vi "DAQmx 9481 Relay (SubVI).vi"(0 "9481 Name":tag="Relay-I", 7 "Relay Control":bool[](array[boolean])=[FALSE, FALSE, FALSE, FALSE], 11 "Error Input":errorcluster, 14 "Stop Program":bool) -> (15 "Relay Error":errorcluster)   [LabVIEW 2011]
uses:
  <vilib>/DAQmx/write.llb/DAQmx Write (Digital 1D Bool NChan 1Samp 1Line).vi
  <vilib>/DAQmx/create/channels.llb/DAQmx Create Channel (DO-Digital Output).vi
  <vilib>/DAQmx/miscellaneous.llb/DAQmx Fill In Error Info.vi
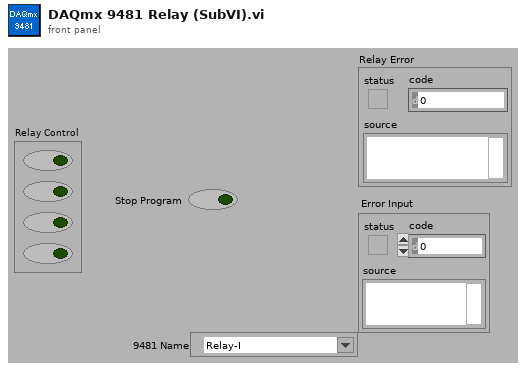
[diagram p1: front panel]
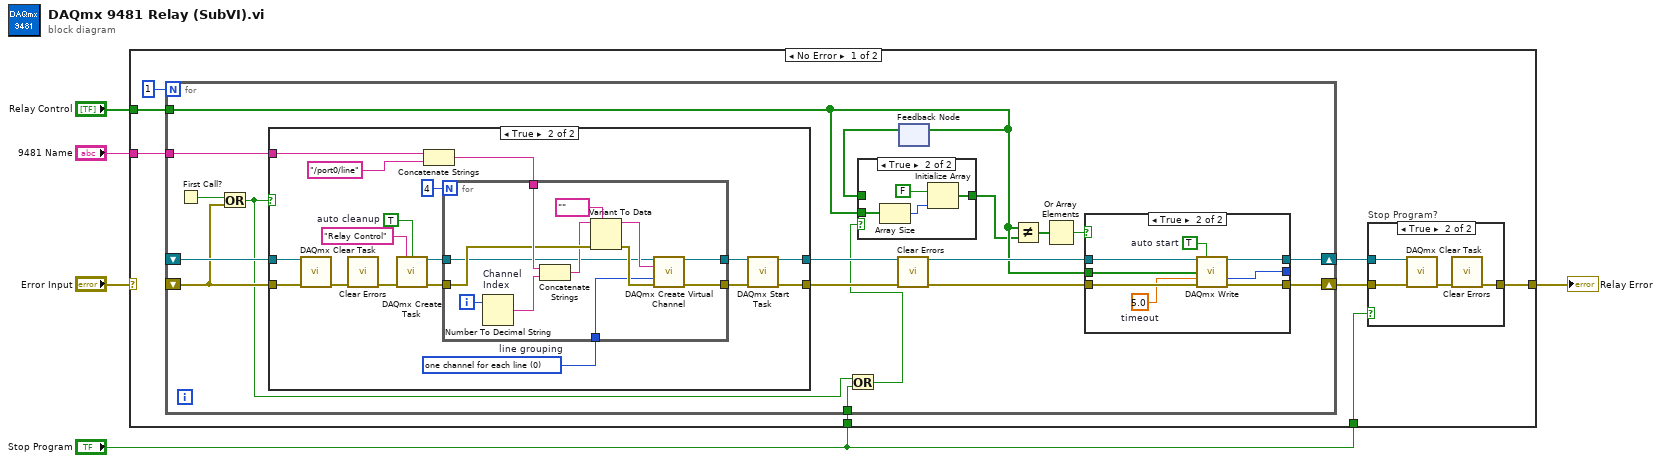
[diagram p0: block diagram]
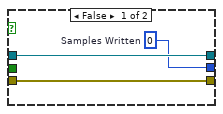
[diagram p3: hidden frame]
diagram:
  n1 = case shown="No Error" "Error Input" {
    selector: "Error Input" -> [_ w83]
    tunnel: "Relay Control" -> [w13 _]
    tunnel: [w12 w83] -> w4
    tunnel: "Stop Program" -> [w9 _]
    tunnel: "9481 Name" -> [w7 _]
    tunnel: "Stop Program" -> [w6 _]
    frame No Error {
      n2 = for {
        N: 1 -> [_]
        tunnel: w13 -> [w29]
        shift-right: [w27] -> w10
        shift-left: _ -> [w26]
        shift-right: [w28] -> w11
        shift-left: _ -> [w17]
        tunnel: w7 -> [w24]
        tunnel: w6 -> [w14]
        n3 = First Call?() -> (First Call?: T/F=w25:bool)
        n4 = Or(x=w25, y=w17) -> (x .or. y?=w16:bool)
        n5 = case shown="True" w16 {
          tunnel: [w48 w54] -> w30
          tunnel: [w47 w53] -> w19
          tunnel: w17 -> [w47 w58]
          tunnel: w26 -> [w48 w59]
          tunnel: w24 -> [_ w52]
          frame False {
          }
          frame True {
            w63 = 0 items=["one channel for each line", "one channel for all lines"]  # line grouping
            w65 = TRUE  # auto cleanup
            n6 = call <vilib>:"DAQmx Clear Task.vi"("task in"=w59, "error in"=w58) -> ("error out"=w57:errorcluster)  [unwired: 13 in]
            n7 = call <vilib>:"Clear Errors.vi"("error in (no error)"=w57) -> ("error out"=w56:errorcluster)  [unwired: 6 in]
            n8 = call <vilib>:"DAQmx Create Task.vi"("new task name"="Relay Control", "auto cleanup"=w65, "error in"=w56) -> ("task out"=w61:refnum<k21>, "error out"=w62:errorcluster)  [unwired: 11 in]
            n9 = Concatenate Strings(w52, "/port0/line" ("string")) -> (w51:string)
            n10 = for {
              N: 4 -> [_]
              tunnel: w51 -> [w75]
              tunnel: w62 -> [w73]
              tunnel: [w67] -> w49
              tunnel: w61 -> [w69]
              tunnel: [w68] -> w50
              tunnel: w63 -> [w66]
              i -> [w76]
              n11 = Number To Decimal String "Channel\nIndex"(number=w76) -> (decimal integer string=w77:string)  [unwired: 1 in]
              n12 = Concatenate Strings(w75, w77) -> (w70:string)
              n13 = Variant To Data(error in=w73, type=tag "" ("physical channels"), Variant=w70) -> (data=w71:tag, error out=w72:errorcluster)
              n14 = call-poly <vilib>:"DAQmx Create Virtual Channel.vi"("task in"=w69, "lines"=w71, "line grouping"=w66, "error in"=w72) -> ("task out"=w68:refnum<k21>, "error out"=w67:errorcluster)  [unwired: 10 in]
            }
            n15 = call <vilib>:"DAQmx Start Task.vi"("task/channels in"=w50, "error in"=w49) -> ("task out"=w54:refnum<k21>, "error out"=w53:errorcluster)  [unwired: 12 in]
          }
        }
        n16 = Or(x=w16, y=w14) -> (x .or. y?=w15:bool)
        n17 = call <vilib>:"Clear Errors.vi"("error in (no error)"=w19) -> ("error out"=w18:errorcluster)  [unwired: 6 in]
        n18 = feedback #1() -> (w21:bool[])  [unwired: 1 in]
        n19 = case shown="True" w15 {
          tunnel: w29 -> [_ w33]
          tunnel: [w31 w32] -> w20
          tunnel: w21 -> [w31 _]
          frame False {
          }
          frame True {
            n20 = Array Size(array=w33) -> (size(s)=w34:i32)
            n21 = Initialize Array(FALSE, w34) -> (w32:bool[])
          }
        }
        n22 = feedback-in #1(w29) -> ()
        n23 = Not Equal?(x=w29, y=w20) -> (x != y?=w23:bool[])
        n24 = Or Array Elements(Boolean array=w23) -> (logical OR=w22:bool)
        n25 = case shown="True" w22 {
          tunnel: w30 -> [w38 w45]
          tunnel: w18 -> [w36 w44]
          tunnel: w29 -> [_ w43]
          tunnel: [w36 w42] -> w28
          tunnel: [w37 w40] -> _
          tunnel: [w38 w39] -> w27
          frame False {
            w37 = u32 0  # Samples Written
          }
          frame True {
            w41 = 5.0  # timeout
            w46 = TRUE  # auto start
            n26 = call-poly <vilib>:"DAQmx Write.vi"("task/channels in"=w45, "auto start"=w46, "data"=w43, "timeout"=w41, "error in"=w44) -> ("task out"=w39:refnum<k21>, "number of samples written per channel"=w40:u32, "error out"=w42:errorcluster)  [unwired: 8 in]
          }
        }
      }
      n27 = case "Stop Program?" shown="True" w9 {
        tunnel: w10 -> [_ w80]
        tunnel: w11 -> [w78 w81]
        tunnel: [w78 w79] -> w12
        frame False {
        }
        frame True {
          n28 = call <vilib>:"DAQmx Clear Task.vi"("task in"=w80, "error in"=w81) -> ("error out"=w82:errorcluster)  [unwired: 13 in]
          n29 = call <vilib>:"Clear Errors.vi"("error in (no error)"=w82) -> ("error out"=w79:errorcluster)  [unwired: 6 in]
        }
      }
    }
    frame Error {
    }
  }
  "Relay Error" <- w4
